vi "Config Flatten.vi"(8 "error in (no error)":errorcluster, 11 "launcher in":refnum<class "launcher.lvclass">) -> (0 "error out":errorcluster, 2 "Raw Config":string, 3 "launcher out":refnum<class "launcher.lvclass">)   [LabVIEW 2021, in "launcher.lvclass"]
uses:
  launcher.lvclass
  launcher.lvclass/launcher.ctl
  17a77c9b-a3da-4683-a802-7e6901ba3513.vi
  Accessors/Read _PARMS.vi
  <vilib>/JDP Science/JSONtext/Variant to JSON Text.vi
  <vilib>/JDP Science/JSONtext/LVClass Serializer/JSONtext LVClass Serializer.lvclass
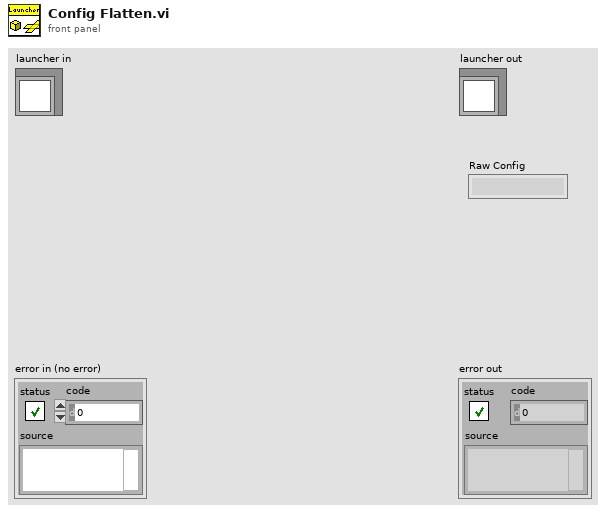
[diagram p1: front panel]
types:
  T1 = typedef "launcher.lvclass/_PARMS.ctl" = cluster{"ch_alias":string[], "ch_units":string[], "Modules to Launch":T2[]}
  T2 = typedef "Module.lvclass/Launch Module Typdef.ctl" = cluster{"Module":string, "Parameters":T3}
  T3 = typedef "Module.lvclass/Launch Module Parms.ctl" = cluster{"Name":string, "Arguments":string[], "Show FP?":bool}
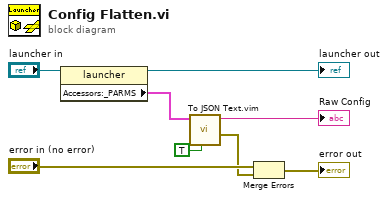
[diagram p0: block diagram]
diagram:
  n1 = property class="launcher"(reference="launcher in") -> (reference out=→"launcher out":refnum<class "launcher.lvclass">, "Accessors:_PARMS"=w1:T1)  [unwired: 1 in, 1 out]
  n2 = call "To JSON Text.vim"("Pretty Print?"=TRUE, "Anything"=w1) -> ("error out"=w6:errorcluster, "<JSON>"=→"Raw Config":string)  [unwired: 8 in]
  n3 = Merge Errors("error in (no error)", w6) -> (→"error out":errorcluster)
